vi "Sets and Query the Temperature Simulation Value.vi"(5 "Enable to Query":bool=TRUE, 7 "Enable to Sets":bool=TRUE, 8 "error in":errorcluster, 10 "Simulation Value":dbl=23.0 min=0.0 max=50.0 step=0.01 format="%#.2f", 11 "VISA resource name":refnum<visa-resource-name>) -> (0 "error out":errorcluster, 2 "Return the Simulation Value":string, 3 "VISA resource name out":refnum<visa-resource-name>)   [LabVIEW 2011, in "DMM4.lvlib"]
uses:
  <instrlib>/DMM4/DMM4.lvlib
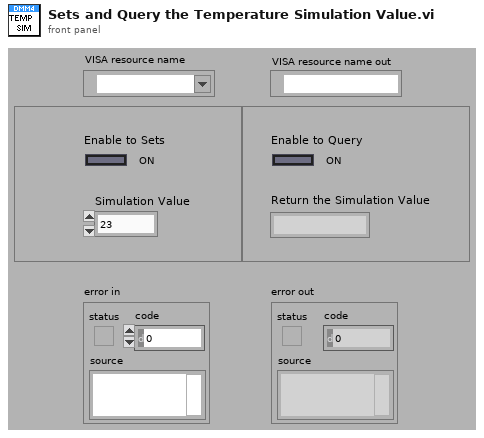
[diagram p1: front panel]
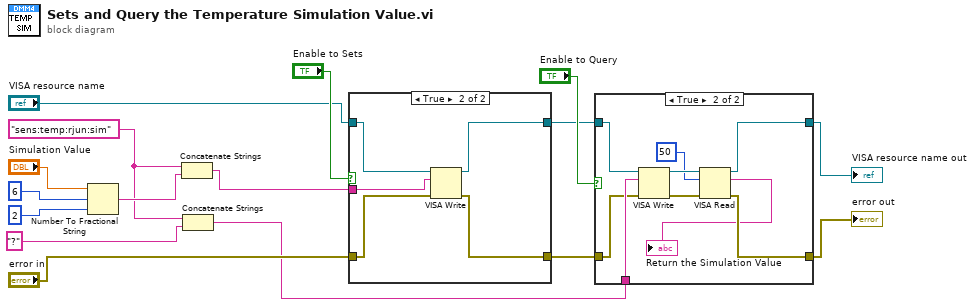
[diagram p0: block diagram]
diagram:
  w11 = "sens:temp:rjun:sim"
  n1 = Number To Fractional String(number="Simulation Value", width (-)=i16 6, precision (6)=i16 2) -> (F-format string=w12:string)  [unwired: 1 in]
  n2 = Concatenate Strings(w11, w12) -> (w7:string)
  n3 = Concatenate Strings(w11, "?") -> (w6:string)
  n4 = case shown="True" "Enable to Sets" {
    tunnel: "VISA resource name" -> [w18 w23]
    tunnel: "error in" -> [w17 w22]
    tunnel: [w18 w21] -> w4
    tunnel: [w17 w20] -> w3
    tunnel: w7 -> [_ w19]
    frame False {
    }
    frame True {
      n5 = VISA Write(VISA resource name=w23, write buffer=w19, error in (no error)=w22) -> (VISA resource name out=w21:refnum<visa-resource-name>, error out=w20:errorcluster)  [unwired: 1 out]
    }
  }
  n6 = case shown="True" "Enable to Query" {
    tunnel: w6 -> [_ w32]
    tunnel: w4 -> [w25 w31]
    tunnel: w3 -> [w24 w30]
    tunnel: [w25 w29] -> w2
    tunnel: [w24 w28] -> w1
    frame False {
    }
    frame True {
      n7 = VISA Write(VISA resource name=w31, write buffer=w32, error in (no error)=w30) -> (VISA resource name out=w33:refnum<visa-resource-name>, error out=w34:errorcluster)  [unwired: 1 out]
      n8 = VISA Read(VISA resource name=w33, byte count=u32 50, error in (no error)=w34) -> (VISA resource name out=w29:refnum<visa-resource-name>, read buffer=→"Return the Simulation Value":string, error out=w28:errorcluster)  [unwired: 1 out]
    }
  }
  "VISA resource name out" <- w2
  "error out" <- w1
